vi "Check and Get Scalar.vi"(8 "error in (no error)":errorcluster, 9 "test commands":string[](array[string]), 10 "variable name":string, 11 "GOLPI ref. in":T1={"pipe handle"={"lv_proc.dll file path"=path "", "process instance handle"=[]}, "fast read timeout [ms]"=500, "fast read settle time [ms]"=10, "fast read to multiple [ms]"=1, "max elements per input line"=100, "slow read timeout [ms]"=5000}) -> (0 "error out":errorcluster, 1 "variable":string, 2 "all tests OK?":bool, 3 "GOLPI ref. out":T1={"pipe handle"={"lv_proc.dll file path"=path "", "process instance handle"=[]}, "fast read timeout [ms]"=500, "fast read settle time [ms]"=10, "fast read to multiple [ms]"=1, "max elements per input line"=100, "slow read timeout [ms]"=5000})   [LabVIEW 2013, in "GOLPI library.lvlib"]
doc: "Checks scalar variable and gets it from GNU Octave in one write-read cycle. 'variable name' is the name of the variable. 'test commands' is array of GNU Octave commands with boolean output applied to the variable. I.e. to read noncomplex double scalar variable 'x', following array should be supplied:\nisnumeric\nisscalar\n~isscomplex\nTests performed are:\nisnumeric(x)\nisscalar(x)\n~iscomplex(x)\nIf output of all tests is '1', output 'all tests OK?' is true."
uses:
  GOLPI library.lvlib
  Type Definitions/GOLPI reference Type Def.ctl
  LV Process.lvlibp/Pipe Handle.ctl
  Type Definitions/Custom Error Codes Enum Type Def.vi
  LV Process.lvlibp
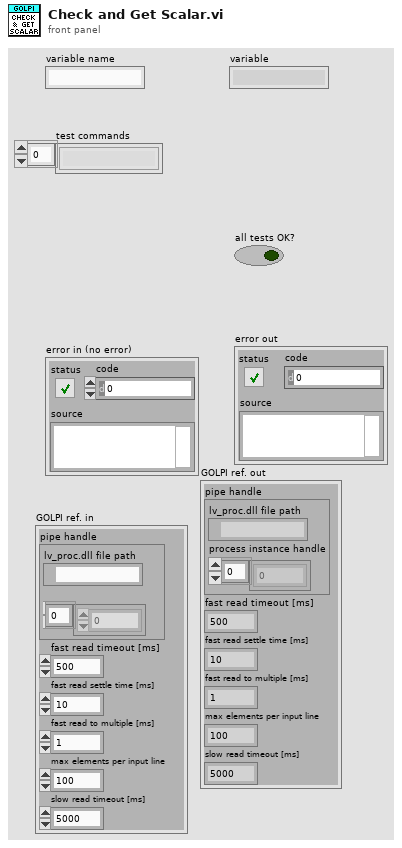
[diagram p1: front panel]
types:
  T1 = typedef "GOLPI library.lvlib/GOLPI reference Type Def.ctl" = cluster{"pipe handle":T2, "fast read timeout [ms]":u32, "fast read settle time [ms]":u32, "fast read to multiple [ms]":u32, "max elements per input line":u32, "slow read timeout [ms]":u32}
  T2 = typedef "LV Process.lvlibp/Pipe Handle.ctl" = cluster{"lv_proc.dll file path":path, "process instance handle":u32[]}
  T3 = typedef "GOLPI library.lvlib/Custom Error Codes Enum Type Def.vi" = enum16{"no error", "00 working directory PAR1 missing", "01 octave binary PAR1 missing", "02 octave report error PAR1", "03 empty output last cmd PAR1", "04 missing temporary file PAR1", "05 pwd PAR 1 not exist", "10 var PAR1 not string", "11 var PAR1 not num, scal, ~compl", "12 var PAR1 not num, scal, compl", "13 var PAR1 not num, vect, ~compl", "14 var PAR1 not num, vect, compl", "15 var PAR1 not num, mat, ~compl", "16 var PAR1 not num, mat, ~compl", "30 WARNING read timeout", "99 not finished"}
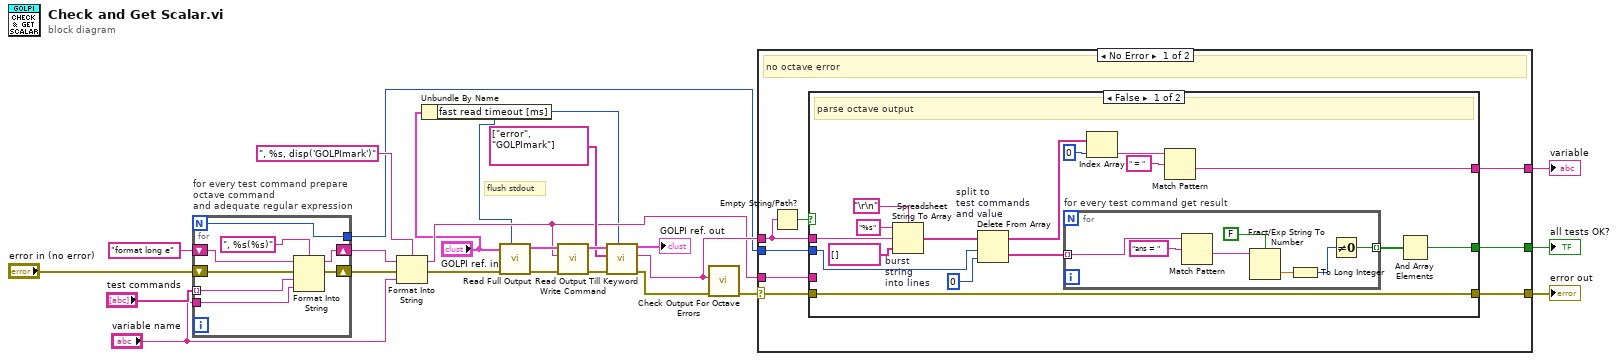
[diagram p0: block diagram]
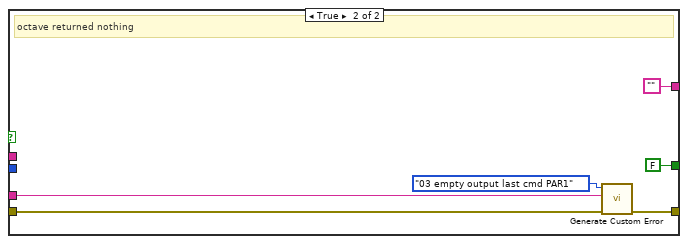
[diagram p2: hidden frame]
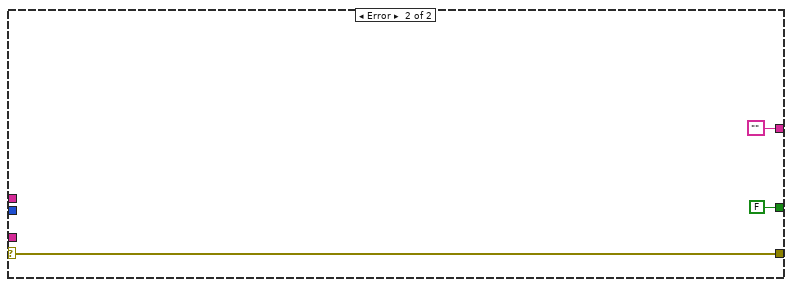
[diagram p3: hidden frame]
diagram:
  # "flush stdout"
  n1 = for "for every test command prepare\noctave command\nand adequate regular expression" {
    N -> [w25]
    tunnel: "test commands" -> [w30] mode=indexing
    tunnel: "variable name" -> [w29]
    shift-right: [w28] -> w5
    shift-left: "format long e" -> [w31]
    shift-right: [w26] -> w18
    shift-left: "error in (no error)" -> [w27]
    tunnel: [w25] -> w4
    n2 = Format Into String(format string=", %s(%s)", initial string=w31, error in=w27, w30, w29) -> (resulting string=w28:string, error out=w26:errorcluster)
  }
  n3 = Format Into String(format string=", %s, disp('GOLPImark')", initial string=w5, error in=w18, "variable name") -> (resulting string=w6:string, error out=w13:errorcluster)
  n4 = Unbundle By Name("GOLPI ref. in") -> ("fast read timeout [ms]"=w2:u32)
  n5 = call "Read Full Output.vi"("timeout [ms]"=w2, "error in"=w13, "GOLPI ref. in"="GOLPI ref. in") -> ("error out"=w14:errorcluster, "GOLPI ref. out"=w15:T1)  [unwired: 5 in, 2 out]
  n6 = call "Write Command.vi"("error in"=w14, "command"=w6, "GOLPI ref. in"=w15) -> ("error out"=w12:errorcluster, "GOLPI ref. out"=w9:T1)  [unwired: 7 in]
  n7 = call "Read Output Till Keyword.vi"("timeout [ms]"=w2, "error in"=w12, "keywords"=string[] ["error", "GOLPImark"], "GOLPI ref. in"=w9) -> ("error out"=w11:errorcluster, "read buffer"=w10:string, "GOLPI ref. out"=→"GOLPI ref. out":T1)  [unwired: 4 in, 1 out]
  n8 = call "Check Output For Octave Errors.vi"("error in"=w11, "read buffer"=w10) -> ("error out"=w7:errorcluster)  [unwired: 9 in]
  n9 = case shown="No Error" w7 {
    selector: w7 -> [w36 w72]
    tunnel: [w40 ""] -> w20
    tunnel: [w39 FALSE] -> w19
    tunnel: [w38 w72] -> w17
    tunnel: w10 -> [w37 _]
    tunnel: w6 -> [w34 _]
    tunnel: w4 -> [w33 _]
    frame No Error {
      # "no octave error"
      n10 = Empty String/Path?(string/path=w37) -> (empty?=w35:bool)
      n11 = case shown="False" w35 {
        tunnel: [w41 ""] -> w40
        tunnel: [w49 FALSE] -> w39
        tunnel: [w48 w64] -> w38
        tunnel: w37 -> [w47 _]
        tunnel: w36 -> [w48 w65]
        tunnel: w34 -> [_ w66]
        tunnel: w33 -> [w46 _]
        frame False {
          # "parse octave output"
          n12 = Spreadsheet String To Array "burst\nstring\ninto lines"(delimiter (Tab)="\r\n", format string="%s", spreadsheet string=w47, array type (2D Dbl)=string[] []) -> (array=w53:string[])
          n13 = Delete From Array "split to\ntest commands\nand value"(array=w53, length=w46, index=0) -> (deleted portion=w55:string[], array with subset deleted=w44:string[])
          n14 = for "for every test command get result" {
            tunnel: w55 -> [w63] mode=indexing
            tunnel: [w57] -> w56 mode=indexing
            n15 = Match Pattern(string=w63, regular expression="ans = ") -> (after substring=w59:string)  [unwired: 1 in, 3 out]
            n16 = Fract/Exp String To Number(use system decimal point (T)=FALSE, string=w59) -> (number=w60:dbl)  [unwired: 2 in, 1 out]
            n17 = To Long Integer(number=w60) -> (32bit integer=w61:i32)
            n18 = Not Equal To 0?(x=w61) -> (x != 0?=w57:bool)
          }
          n19 = Index Array(array=w44, index=0) -> (element=w42:string)
          n20 = Match Pattern(string=w42, regular expression=" = ") -> (after substring=w41:string)  [unwired: 1 in, 3 out]
          n21 = And Array Elements(Boolean array=w56) -> (logical AND=w49:bool)
        }
        frame True {
          # "octave returned nothing"
          n22 = call "Generate Custom Error.vi"("error in"=w65, "PAR1"=w66, "GOLPI error"=Custom_Error_Codes_Enum_Type_Def.vi."03 empty output last cmd PAR1" ("Enum")) -> ("error out"=w64:errorcluster)  [unwired: 8 in]
        }
      }
    }
    frame Error {
    }
  }
  "all tests OK?" <- w19
  "variable" <- w20
  "error out" <- w17
